vi "OpnCrtRep File.vi"(4 "advisory dialog? (display:T)":bool=TRUE, 5 "file dialog info":T1={"prompt"="", "pattern"="", "default name"="", "start path"=path ""}, 7 "function (open:0)":T4(ring), 8 "error in":errorcluster, 9 "deny mode (2)":T2(ring)=enum."deny none", 10 "open mode (0)":T3(ring), 11 "file path":path) -> (0 "error out":errorcluster, 1 "file size (bytes)":i32, 2 "new file path":path, 3 "refnum":refnum<file>)   [LabVIEW 2012, in "Car Wash.lvlib" / "Tools_String.lvlib"]
doc: "This VI is the same as the \"Open/Create/Replace File.vi\" except that it allows you to specify the open and deny modes. It passes the information for the file dialog as a cluster instead of individual parameters.\n\nOpens an existing file, creates a new file, or replaces an existing file, programmatically or interactively using dialog. You can optionally specify a dialog prompt, default file name, start path, or filter pattern, and you can specify open and deny modes when opening a file, plus group and permission when creating a new file. Use this VI with the intermediate Write File+ or Read File+ VIs described below.\n\nfile path is the path name of the file. If file path is empty (default value) or is Not A Path, the VI displays a File dialog box from which you can select a file. Error 43 occurs if the user cancels the dialog. \n\nfunction is the operation to perform:\n\n 0 (open) opens an existing file. Error 7 occurs if the file cannot be found.\n \n 1 (open or create) opens an existing file or creates a new file if one does not exist.\n\n 2 (create or replace) creates a new file or replaces a file if it exists and you give permission. Replacement is done by opening the file and setting EOF to 0. Error 43 occurs if the user elects to disallow the replacement using dialog. \n\n 3 (create) creates a new file. Error 8 occurs if the file already exists.\n\nadvisory dialog? Set TRUE (default) if you want a dialog if function=0 and the file does not exist, or if function=2 or 3 and the file exists.\n\nprompt is the message that appears below the list of files and directories in the file dialog.\n\ndefault name is the initial file name that appears in the selection box of the file dialog.\n\nstart path is the path name to the initially displayed directory in a file dialog. The default value is Not A Path, which is the path to the last directory shown in a file dialog.\n\npattern is the match pattern specification to display only certain types of files or directories. See the description of the File Dialog function for more information.\n\nerror in is a cluster of three elements (error?, code, and source) that describe the upstream error state, that is, the existance of any error preceeding the execution of the VI. The VI executes normally only if no incoming error exists; otherwise it merely passes the error in value to error out. error? is TRUE if an error occurred; the default value is FALSE. code is the error code; the default value is 0. source is in most cases the name of the VI or function that produced the error; the default value is an empty string.\n\nnew file path is the path of the file opened or created. You can use this output to determine the path of a file that you open or create using dialog. new file path returns Not A Path if the user selects Cancel from the dialog box.\n\nrefnum is the reference number of the open file. The value is Not A Refnum if the file cannot be opened.\n\nfile size is the size of the file in bytes; it is also the location of the end of file.\n\nerror out is a cluster of three elements (error?, code, and source) that describe the error state following the execution of the VI. If an incoming error does not exist, the VI executes normally and error out describes the VI's error state; if an incoming error exists, error out equals error in."
uses:
  Tools_String.lvlib
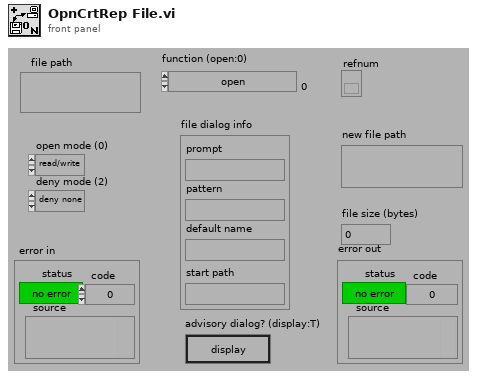
[diagram p1: front panel]
types:
  T1 = cluster{"prompt":string, "pattern":string, "default name":string, "start path":path}
  T2 = enum16{"deny read/write", "deny write-only", "deny none"}
  T3 = enum16{"read/write", "read-only", "write-only", "write-only (truncate)"}
  T4 = enum16{"open", "open or create", "create or replace", "create"}
  T5 = enum16{"open", "replace", "create", "open or create", "replace or create", "replace or create with confirmation"}
  T6 = enum16{"existing file", "new file", "new or existing file", "existing dir", "new dir", "new or existing dir"}[]
  T7 = enum16{"existing file", "new file", "new or existing file", "existing dir", "new dir", "new or existing dir"}
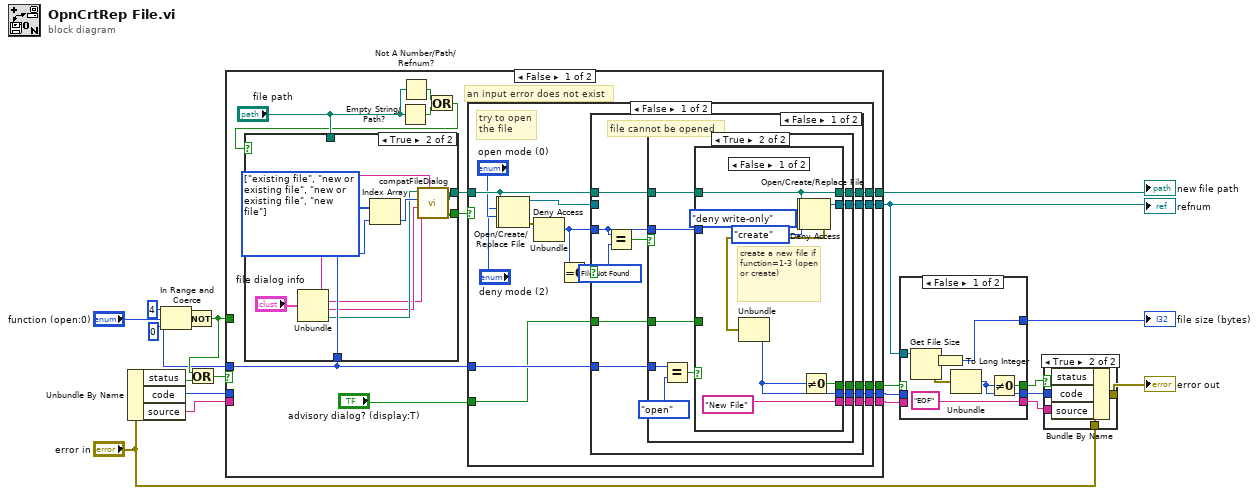
[diagram p0: block diagram]
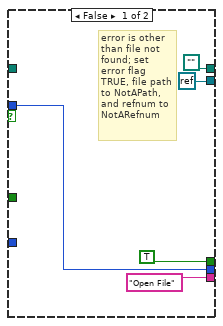
[diagram p4: hidden frame]
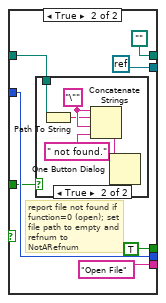
[diagram p5: hidden frame]
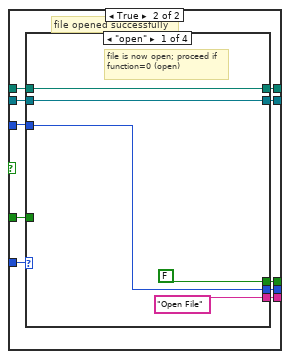
[diagram p7: hidden frame]
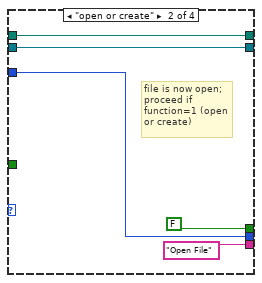
[diagram p8: hidden frame]
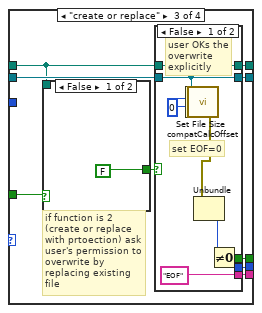
[diagram p9: hidden frame]
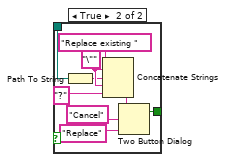
[diagram p10: hidden frame]
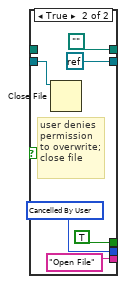
[diagram p11: hidden frame]
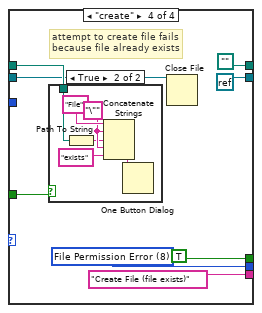
[diagram p12: hidden frame]
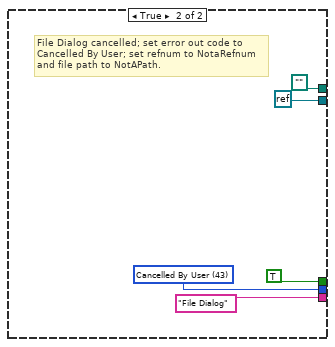
[diagram p14: hidden frame]
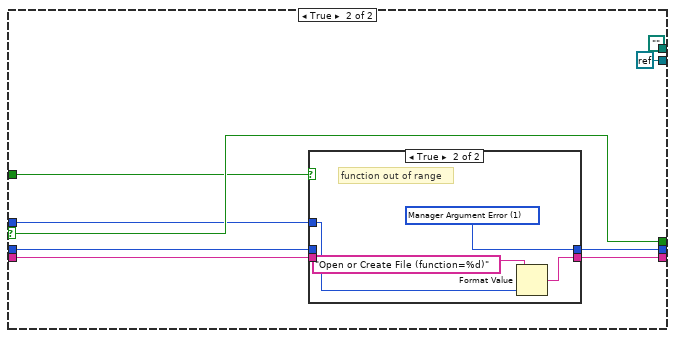
[diagram p16: hidden frame]
diagram:
  n1 = Unbundle By Name("error in") -> ("status"=w10:bool, "code"=w9:i32, "source"=w8:string)
  n2 = In Range and Coerce(upper limit=4, x="function (open:0)", lower limit=0) -> (In Range?=w15:bool)  [unwired: 1 out]
  n3 = Not(x=w15) -> (.not. x?=w17:bool)
  n4 = Or(x=w17, y=w10) -> (x .or. y?=w16:bool)
  n5 = case shown="False" w16 {
    selector: w16 -> [_ w191]
    tunnel: [w31 path ""] -> w20
    tunnel: [w30 refnum<k0> refnum] -> w11
    tunnel: [w29 w188] -> w12
    tunnel: [w28 w191] -> w14
    tunnel: [w27 w190] -> w13
    tunnel: w9 -> [_ w189]
    tunnel: w8 -> [_ w187]
    tunnel: "function (open:0)" -> [w21 w186]
    tunnel: w17 -> [_ w185]
    frame False {
      # "an input error does not exist"
      n6 = Empty String/Path?(string/path="file path") -> (empty?=w24:bool)
      n7 = Not A Number/Path/Refnum?(number/path/refnum="file path") -> (NaN/Path/Refnum?=w25:bool)
      n8 = Or(x=w25, y=w24) -> (x .or. y?=w23:bool)
      n9 = case shown="True" w23 {
        selector: w23 -> [w173 _]
        tunnel: [w173 w184] -> w33
        tunnel: [w174 w183] -> w32
        tunnel: "file path" -> [w174 _]
        tunnel: w21 -> [_ w179]
        frame False {
          # "a File Path is supplied (not empty); proceed"
        }
        frame True {
          w180 = T6 [enum."existing file", enum."new or existing file", enum."new or existing file", enum."new file"] items=["existing file", "new file", "new or existing file", "existing dir", "new dir", "new or existing dir"]
          n10 = Unbundle("file dialog info") -> ("prompt"=w182:string, "pattern"=w175:string, "default name"=w176:string, "start path"=w177:path)
          n11 = Index Array(array=w180, index=w179) -> (element=w181:T7)
          n12 = call <vilib>:"compatFileDialog.vi"("prompt"=w182, "pattern"=w175, "default name"=w176, "select mode (2)"=w181, "start path"=w177) -> ("cancelled"=w184:bool, "path"=w183:path)  [unwired: 2 in, 3 out]
        }
      }
      n13 = case shown="False" w33 {
        tunnel: w32 -> [w48 _]
        tunnel: [w47 path ""] -> w31
        tunnel: w21 -> [w46 _]
        tunnel: [w45 refnum<k0> refnum] -> w30
        tunnel: [w43 "File Dialog"] -> w29
        tunnel: [w42 TRUE] -> w28
        tunnel: [w41 w171] -> w27
        tunnel: "advisory dialog? (display:T)" -> [w39 _]
        frame False {
          # "try to open the file"
          n14 = Open/Create/Replace File(file path (use dialog)=w48, access (0:read/write)="open mode (0)") -> (refnum out=w34:refnum<file>, error out=w35:errorcluster)  [unwired: 1 in, 4 out]
          n15 = Deny Access(4:w35, 6:"deny mode (2)", 7:w34) -> (0:w49:errorcluster, 3:w44:refnum<file>)
          n16 = Unbundle(w49) -> ("code"=w38:i32)  [unwired: 2 out]
          n17 = Equal To 0?(x=w38) -> (x = 0?=w40:bool)
          n18 = case shown="False" w40 {
            tunnel: w38 -> [w51 w101]
            tunnel: w48 -> [w58 w107]
            tunnel: [w57 w108] -> w47
            tunnel: w46 -> [w56 w100]
            tunnel: [w55 w106] -> w45
            tunnel: w44 -> [_ w105]
            tunnel: [w54 w104] -> w43
            tunnel: [w53 w103] -> w42
            tunnel: [w52 w102] -> w41
            tunnel: w39 -> [w50 w99]
            frame False {
              w60 = u16 7 items=["No Error", "Manager Argument Error", "Memory Full", "Out of Zone", "End of File", "File Already Open", "Generic File IO Error", "File Not Found", "File Permission Error", "Disk Full", "Duplicate Path", "Too Many Files Open", "Not Enabled", "Resource File Not Found", "Cannot Add Resource", "Resource Not Found", "Image Not Found", "Image Memory Error", "Pen Does Not Exist", "Config Bad Type", "Config Token Not Found", "Config Parse Error", "Config Memory Error", "Bad External Code Format", "Bad External Code Offset", "External Code Not Present", "Null Window", "Destroy Window Mixup", "Null Menu", "Print Aborted", "Bad Print Record", "Print Driver Error", "Windows Error During Print", "Memory Error During Print", "Print Dialog Error", "Generic Print Error", "Invalid Device Refnum", "Device Not Found", "Device Parameter Error", "Device Unit Error", "Can't Open Device", "Device Call Aborted", "Generic Error", "Cancelled By User"]
              # "file cannot be opened"
              n19 = Equal?(x=w51, y=w60) -> (x = y?=w59:bool)
              n20 = case shown="True" w59 {
                tunnel: w58 -> [_ w76]
                tunnel: [path "" w75] -> w57
                tunnel: w56 -> [_ w68]
                tunnel: [refnum<k0> refnum w74] -> w55
                tunnel: ["Open File" w73] -> w54
                tunnel: [TRUE w72] -> w53
                tunnel: [w61 w71] -> w52
                tunnel: w51 -> [w61 w70]
                tunnel: w50 -> [_ w69]
                frame False {
                  # "error is other than file not found; set error flag TRUE, file path to NotAPath, and refnum to NotARefnum"
                }
                frame True {
                  n21 = Equal?(x=w68, y=T4."open") -> (x = y?=w67:bool)
                  n22 = case shown="False" w67 {
                    tunnel: w76 -> [w86 w90]
                    tunnel: [w86 path ""] -> w75
                    tunnel: [w85 refnum<k0> refnum] -> w74
                    tunnel: ["New File" "Open File"] -> w73
                    tunnel: [w84 TRUE] -> w72
                    tunnel: [w81 w91] -> w71
                    tunnel: w70 -> [_ w91]
                    tunnel: w69 -> [_ w87]
                    frame False {
                      # "create a new file if function=1-3 (open or create)"
                      n23 = Open/Create/Replace File(file path (use dialog)=w86, operation (0:open)=T5."create") -> (refnum out=w78:refnum<file>, error out=w79:errorcluster)  [unwired: 1 in, 4 out]
                      n24 = Deny Access(4:w79, 6:T2."deny write-only", 7:w78) -> (0:w83:errorcluster, 3:w85:refnum<file>)
                      n25 = Unbundle(w83) -> ("code"=w81:i32)  [unwired: 2 out]
                      n26 = Not Equal To 0?(x=w81) -> (x != 0?=w84:bool)
                    }
                    frame True {
                      # "report file not found if function=0 (open); set file path to empty and refnum to NotARefnum"
                      n27 = case shown="True" w87 {
                        tunnel: w90 -> [_ w94]
                        frame False {
                        }
                        frame True {
                          w96 = "\""
                          n28 = Path To String(path=w94) -> (string=w95:string)
                          n29 = Concatenate Strings(w96, w95, w96, " not found.") -> (w98:string)
                          n30 = One Button Dialog(message=w98) -> ()  [unwired: 2 out]
                        }
                      }
                    }
                  }
                }
              }
            }
            frame True {
              # "file opened successfully"
              n31 = case shown="\"open\"" w100 {
                tunnel: [w113 w114 w127 path ""] -> w108
                tunnel: w107 -> [w113 w114 w119 w161]
                tunnel: [w112 w115 w126 refnum<k0> refnum] -> w106
                tunnel: w105 -> [w112 w115 w125 w158]
                tunnel: ["Open File" "Open File" w124 "Create File (file exists)"] -> w104
                tunnel: [FALSE FALSE w123 TRUE] -> w103
                tunnel: [w109 w117 w122 w159] -> w102
                tunnel: w101 -> [w109 w117 _ _]
                tunnel: w99 -> [_ _ w120 w160]
                frame "open" {
                  # "file is now open; proceed if function=0 (open)"
                }
                frame "open or create" {
                  # "file is now open; proceed if function=1 (open or create)"
                }
                frame "create or replace" {
                  # "if function is 2 (create or replace with prtoection) ask user's permission to overwrite by replacing existing file"
                  n32 = case shown="False" w120 {
                    tunnel: [FALSE w136] -> w121
                    tunnel: w119 -> [_ w129]
                    frame False {
                    }
                    frame True {
                      w131 = "\""
                      n33 = Path To String(path=w129) -> (string=w130:string)
                      n34 = Concatenate Strings("Replace existing ", w131, w130, w131, "?") -> (w137:string)
                      n35 = Two Button Dialog(message=w137, 1:"Replace", 2:"Cancel") -> (T button?=w136:bool)
                    }
                  }
                  n36 = case shown="False" w121 {
                    tunnel: [w142 path ""] -> w127
                    tunnel: [w147 refnum<k0> refnum] -> w126
                    tunnel: w125 -> [w147 w151]
                    tunnel: ["EOF" "Open File"] -> w124
                    tunnel: [w145 TRUE] -> w123
                    tunnel: [w141 w148] -> w122
                    tunnel: w119 -> [w142 _]
                    frame False {
                      w146 = 0
                      # "set EOF=0"
                      # "user OKs the overwrite explicitly"
                      n37 = call <vilib>:"compatCalcOffset.vi"("pos offset (0)"=w146, "pos mode (0:1)"=w146, "refnum"=w147) -> ("error out"=w140:errorcluster, "offset"=w139:i32, "dup refnum"=w138:refnum<file>)  [unwired: 1 in, 5 out]
                      n38 = Set File Size(4:w140, 6:w139, 7:w138) -> (0:w144:errorcluster)  [unwired: 1 out]
                      n39 = Unbundle(w144) -> ("code"=w141:i32)  [unwired: 2 out]
                      n40 = Not Equal To 0?(x=w141) -> (x != 0?=w145:bool)
                    }
                    frame True {
                      w148 = u16 43 items=["No Error", "Manager Argument Error", "Memory Full", "Out of Zone", "End of File", "File Already Open", "Generic File IO Error", "File Not Found", "File Permission Error", "Disk Full", "Duplicate Path", "Too Many Files Open", "Not Enabled", "Resource File Not Found", "Cannot Add Resource", "Resource Not Found", "Image Not Found", "Image Memory Error", "Pen Does Not Exist", "Config Bad Type", "Config Token Not Found", "Config Parse Error", "Config Memory Error", "Bad External Code Format", "Bad External Code Offset", "External Code Not Present", "Null Window", "Destroy Window Mixup", "Null Menu", "Print Aborted", "Bad Print Record", "Print Driver Error", "Windows Error During Print", "Memory Error During Print", "Print Dialog Error", "Generic Print Error", "Invalid Device Refnum", "Device Not Found", "Device Parameter Error", "Device Unit Error", "Can't Open Device", "Device Call Aborted", "Generic Error", "Cancelled By User"]
                      # "user denies permission to overwrite; close file"
                      n41 = Close File(refnum=w151) -> ()  [unwired: 1 in, 2 out]
                    }
                  }
                }
                frame "create" {
                  w159 = u16 8 items=["No Error", "Argument Error", "Memory Full", "Out of Zone", "End of File", "File Already Open", "Generic File IO Error", "File Not Found", "File Permission Error", "Disk Full", "Duplicate Path", "Too Many Files Open", "Not Enabled", "Resource File Not Found", "Cannot Add Resource", "Resource Not Found", "Image Not Found", "Image Memory Error", "Pen Does Not Exist", "Config Bad Type", "Config Token Not Found", "Config Parse Error", "Config Memory Error", "Bad External Code Format", "Bad External Code Offset", "External Code Not Present", "Null Window", "Destroy Window Mixup", "Null Menu", "Print Aborted", "Bad Print Record", "Print Driver Error", "Windows Error During Print", "Memory Error During Print", "Print Dialog Error", "Generic Print Error", "Invalid Device Refnum", "Device Not Found", "Device Parameter Error", "Device Unit Error", "Can't Open Device", "Device Call Aborted", "Generic Error", "Cancelled By User", "Object ID Too Low", "Object ID Too High", "Object Not In Heap", "Unknown Heap", "Bad DefProc ID", "DefProc Not In Table", "Message Out Of Range", "Null Method", "Unknown Message", "Manager Call Not Supported", "Bad address", "Connection In progress", "Connection timed out", "Connection is already in progress", "Network attribute not supported", "Network error", "Address in use", "System out of memory", "Connection aborted", "Connection refused", "Connection is not connected", "Connection is already connected", "Connection closed", "Initialize error (interapplication manager)", "Bad occurrence", "Wait on unbound occurrence handler", "Occurrence queue overflow", "Bad path", "Semaphore not signaled", "Unrecognized type (interapplication manager)"]
                  # "attempt to create file fails because file already exists"
                  n42 = case shown="True" w160 {
                    tunnel: w161 -> [_ w163]
                    frame False {
                    }
                    frame True {
                      w165 = "\""
                      n43 = Path To String(path=w163) -> (string=w164:string)
                      n44 = Concatenate Strings("File", w165, w164, w165, "exists") -> (w162:string)
                      n45 = One Button Dialog(message=w162) -> ()  [unwired: 2 out]
                    }
                  }
                  n46 = Close File(refnum=w158) -> ()  [unwired: 1 in, 2 out]
                }
              }
            }
          }
        }
        frame True {
          w171 = u16 43 items=["No Error", "Manager Argument Error", "Memory Full", "Out of Zone", "End of File", "File Already Open", "Generic File IO Error", "File Not Found", "File Permission Error", "Disk Full", "Duplicate Path", "Too Many Files Open", "Not Enabled", "Resource File Not Found", "Cannot Add Resource", "Resource Not Found", "Image Not Found", "Image Memory Error", "Pen Does Not Exist", "Config Bad Type", "Config Token Not Found", "Config Parse Error", "Config Memory Error", "Bad External Code Format", "Bad External Code Offset", "External Code Not Present", "Null Window", "Destroy Window Mixup", "Null Menu", "Print Aborted", "Bad Print Record", "Print Driver Error", "Windows Error During Print", "Memory Error During Print", "Print Dialog Error", "Generic Print Error", "Invalid Device Refnum", "Device Not Found", "Device Parameter Error", "Device Unit Error", "Can't Open Device", "Device Call Aborted", "Generic Error", "Cancelled By User"]
          # "File Dialog cancelled; set error out code to Cancelled By User; set refnum to NotaRefnum and file path to NotAPath."
        }
      }
    }
    frame True {
      n47 = case shown="True" w185 {
        tunnel: [w195 w199] -> w190
        tunnel: w189 -> [w195 _]
        tunnel: [w194 w198] -> w188
        tunnel: w187 -> [w194 _]
        tunnel: w186 -> [_ w196]
        frame False {
          # "on an input error, do nothing"
        }
        frame True {
          w199 = u16 1 items=["No Error", "Manager Argument Error", "Memory Full", "Out of Zone", "End of File", "File Already Open", "Generic File IO Error", "File Not Found", "File Permission Error", "Disk Full", "Duplicate Path", "Too Many Files Open", "Not Enabled", "Resource File Not Found", "Cannot Add Resource", "Resource Not Found", "Image Not Found", "Image Memory Error", "Pen Does Not Exist", "Config Bad Type", "Config Token Not Found", "Config Parse Error", "Config Memory Error", "Bad External Code Format", "Bad External Code Offset", "External Code Not Present", "Null Window", "Destroy Window Mixup", "Null Menu", "Print Aborted", "Bad Print Record", "Print Driver Error", "Windows Error During Print", "Memory Error During Print", "Print Dialog Error", "Generic Print Error", "Invalid Device Refnum", "Device Not Found", "Device Parameter Error", "Device Unit Error", "Can't Open Device", "Device Call Aborted", "Generic Error", "Cancelled By User"]
          # "function out of range"
          n48 = Format Value(format string="Open or Create File (function=%d)", value (0)=w196) -> (output string=w198:string)  [unwired: 1 out]
        }
      }
    }
  }
  "new file path" <- w20
  "refnum" <- w11
  n49 = case shown="False" w14 {
    selector: w14 -> [_ w209]
    tunnel: w13 -> [_ w208]
    tunnel: w12 -> [_ w207]
    tunnel: [w205 w209] -> w7
    tunnel: [w203 w208] -> w6
    tunnel: ["EOF" w207] -> w5
    tunnel: w11 -> [w204 _]
    tunnel: [w200 _] -> w1
    frame False {
      n50 = Get File Size(file=w204) -> (size (in bytes)=w201:i64, 0:w202:errorcluster)  [unwired: 1 in, 1 out]
      n51 = To Long Integer(number=w201) -> (32bit integer=w200:i32)
      n52 = Unbundle(w202) -> ("code"=w203:i32)  [unwired: 2 out]
      n53 = Not Equal To 0?(x=w203) -> (x != 0?=w205:bool)
    }
    frame True {
    }
  }
  "file size (bytes)" <- w1
  n54 = case shown="True" w7 {
    selector: w7 -> [_ w214]
    tunnel: w6 -> [_ w215]
    tunnel: w5 -> [_ w213]
    tunnel: "error in" -> [w210 w212]
    tunnel: [w210 w211] -> w3
    frame False {
    }
    frame True {
      n55 = Bundle By Name(cluster=w212, "status"=w214, "code"=w215, "source"=w213) -> (w211:errorcluster)
    }
  }
  "error out" <- w3
